vi "AM Modulation Demo (music) - Square.vi"() -> ()   [LabVIEW 2013]
uses:
  <vilib>/sound2/lvsound2.llb/Sound File Info (path).vi
  <vilib>/sound2/lvsound2.llb/Sound File Read Open.vi
  <vilib>/sound2/lvsound2.llb/Sound File Read (DBL).vi
  <vilib>/Waveform/WDTOps.llb/WDT Get Waveform Subset DBL.vi
  <vilib>/express/express analysis/Spectral/Block/exnSpectralBlock spectral measurements RMS poly.vi
  <vilib>/express/express analysis/Spectral/Block/exnSpectralBlock spectral measurements RMS DDT.vi
  <vilib>/express/express analysis/Spectral/Block/exnSpectralBlock spectral measurements power poly.vi
  <vilib>/express/express analysis/Spectral/Block/exnSpectralBlock spectral measurements power DDT.vi
  <vilib>/express/express analysis/Spectral/XNode/ExpressSpectralMeasurementsBlockNode.xnode
panel:
  in  "Duration":dbl
  in  "Path":path
  in  "WAV Sample Rate":dbl=44100.0 caption="dt"
  in  "Resample Rate.":dbl=2000.0 caption="Frequency"
  in  "LPF Cut-Off":dbl=10000.0 caption="Lower Cut-Off"
  in  "SNR (dB)":dbl(slide)=0.6 caption="Standard deviation" scale=-20.0..30.0
  out "Comparision":dynamicdata(graph)
  out "Baseband":dynamicdata(graph)
  out "DSB FFT":dynamicdata(graph)
  out "DSB Signal":dynamicdata(graph)
  out "?":dbl=1.0
  in  "Carrier Amp.":dbl=1.0 caption="Amplitude"
  in  "stop":bool
  in  "Frequency Offset":dbl(slide)=1.0 scale=0.0..1000.0
  in  "Carrier Freq.":dbl=100000.0 caption="Frequency"
  out "DSB Squared":dynamicdata(graph)=[{"t0"=timestamp(0 s since 1904-01-01), "dt"=10.0, "Y"=array[50000 elements], "attributes"=variant("NI_ChannelName"=variant(string "Sine (Power Spectrum)"), "NI_ExpIsRelativeTime"=variant(bool TRUE), "NI_ExpStartTimeStamp"=variant(timestamp timestamp(3635665779.2842293 s since 1904-01-01)), "NI_ExpTimeStamp"=variant(timestamp timestamp(3635665779.2842293 s since 1904-01-01)), "NI_ExpXDimension"=variant(string "f"), "NI_OriginalChannelName"=variant(string "Sine"))}]
  # "Amplitude Modulation"
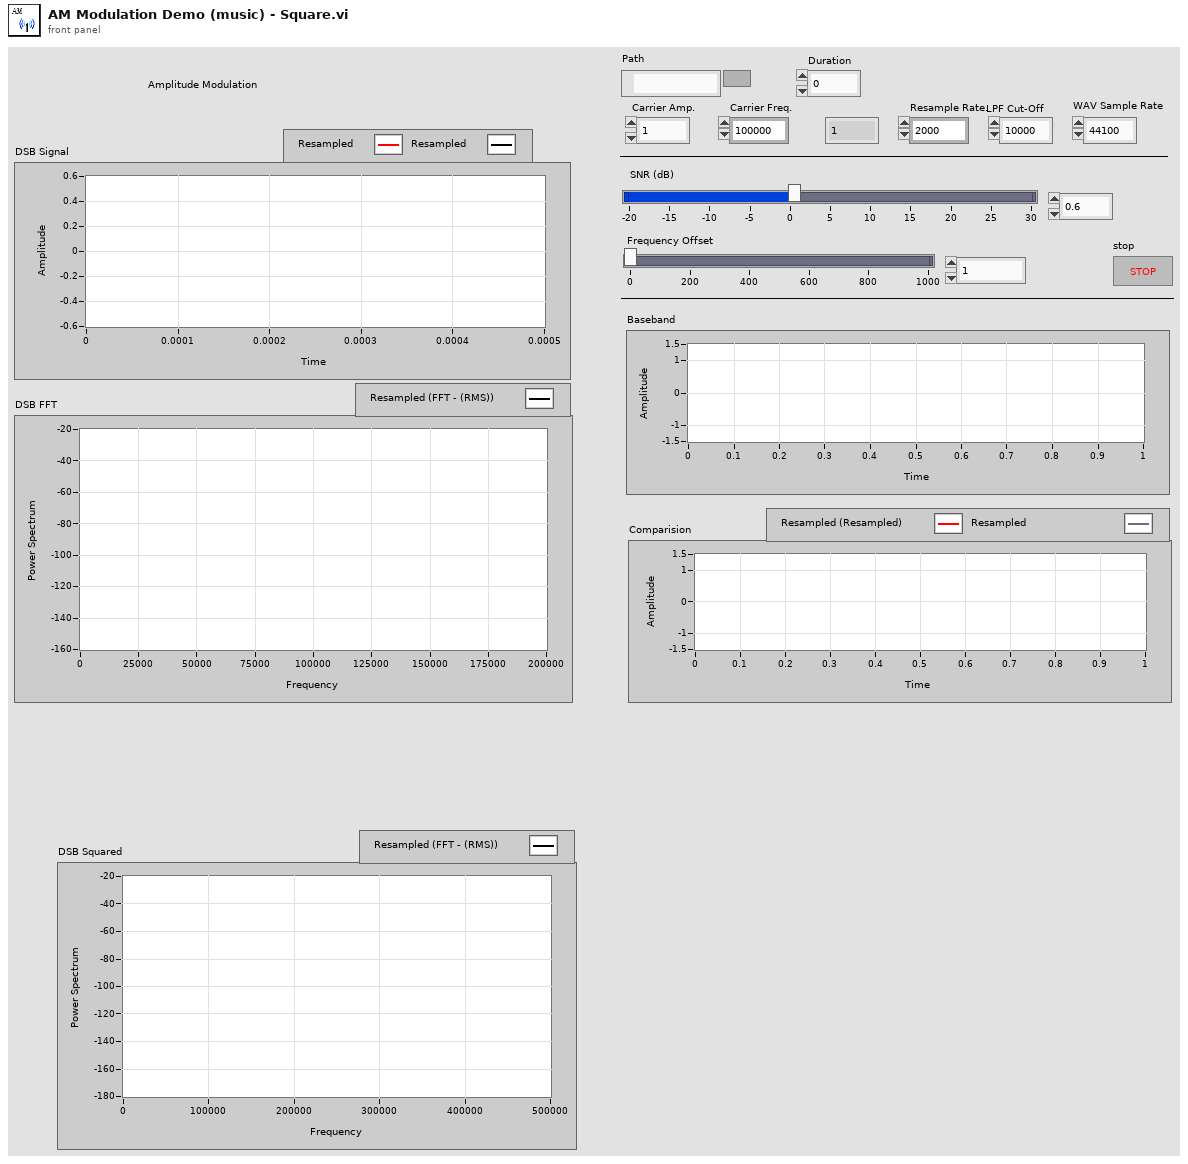
[diagram p1: front panel]
types:
  T1 = typedef "Sound File Refnum.ctl" = refnum<file>
  T2 = cluster{"averaging mode":u16, "weighting mode":u16, "number of averages":u32}
  T3 = cluster{"dB On (F)":bool, "unwrap phase (F)":bool, "convert to degree (F)":bool}
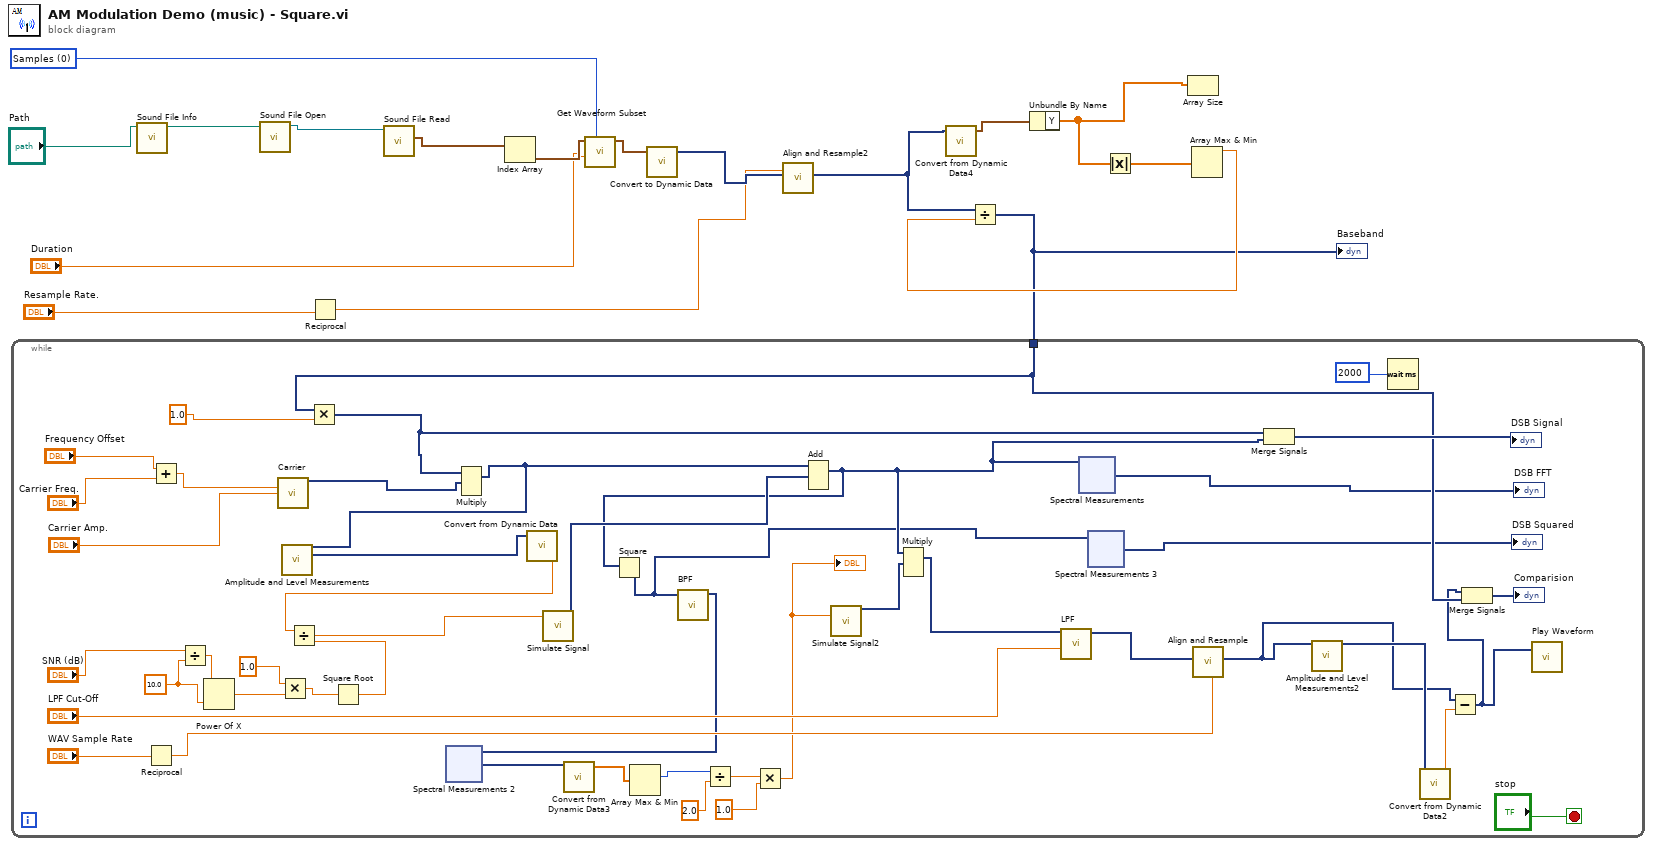
[diagram p0: block diagram]
diagram:
  w12 = u16 0 items=["Samples", "Relative Time"] ("start/duration format")
  n1 = call-poly <vilib>:"Sound File Info.vi"("path"="Path") -> ("path out"=w16:path)  [unwired: 7 in, 3 out]
  n2 = call-poly <vilib>:"Sound File Open.vi"("path"=w16) -> ("sound file refnum"=w15:T1)  [unwired: 9 in, 1 out]
  n3 = Reciprocal(x="Resample Rate.") -> (1/x=w7:dbl)
  n4 = call-poly <vilib>:"Sound File Read.vi"("sound file refnum"=w15) -> ("data"=w14:waveform(dbl)[])  [unwired: 6 in, 4 out]
  n5 = Index Array "Index Array"(array=w14) -> (element=w13:waveform(dbl))  [unwired: 1 in]
  n6 = call-poly <vilib>:"Get Waveform Subset.vi"("start/duration format"=w12, "duration"="Duration", "waveform in"=w13) -> ("waveform out"=w10:waveform(dbl))  [unwired: 3 in, 3 out]
  n7 = call "Convert to Dynamic Data"("Waveform"=w10) -> ("Dynamic Data Type"=w9:dynamicdata)  [unwired: 3 in]
  n8 = call "Align and Resample2"("dt"=w7, "Signals"=w9) -> ("Resampled Signals"=w3:dynamicdata)  [unwired: 7 in, 2 out]
  n9 = call "Convert from Dynamic Data4"("Dynamic Data Type"=w3) -> ("Waveform"=w6:waveform(dbl))  [unwired: 3 in]
  n10 = Unbundle By Name(w6) -> ("Y"=w5:dbl[])
  n11 = Absolute Value(x=w5) -> (abs(x)=w4:dbl[])
  n12 = Array Size(array=w5) -> ()  [unwired: 1 out]
  n13 = Array Max & Min(array=w4) -> (max value=w2:dbl)  [unwired: 3 out]
  n14 = Divide(x=w3, y=w2) -> (x/y=w1:dynamicdata)
  "Baseband" <- w1
  n15 = while {
    tunnel: w1 -> [w45]
    stop <- "stop" stop-if-true
    w41 = 10.0
    n16 = Reciprocal(x="WAV Sample Rate") -> (1/x=w49:dbl)
    n17 = Add(x="Frequency Offset", y="Carrier Freq.") -> (x+y=w34:dbl)
    n18 = Divide(x="SNR (dB)", y=w41) -> (x/y=w42:dbl)
    n19 = Power Of X(1:w41, 2:w42) -> (0:w40:dbl)
    n20 = call "Carrier"("Frequency"=w34, "Amplitude"="Carrier Amp.") -> ("Sine"=w61:dynamicdata)  [unwired: 12 in, 1 out]
    n21 = Multiply(x=1.0, y=w40) -> (x*y=w55:dbl)
    n22 = Multiply(x=w45, y=1.0) -> (x*y=w35:dynamicdata)
    n23 = Square Root(x=w55) -> (sqrt(x)=w53:dbl)
    n24 = Multiply(1:w61, 2:w35) -> (0:w52:dynamicdata)  [unwired: 1 in, 1 out]
    n25 = call "Amplitude and Level Measurements"("Signals"=w52) -> ("RMS"=w59:dynamicdata)  [unwired: 13 in, 1 out]
    n26 = call "Convert from Dynamic Data"("Dynamic Data Type"=w59) -> ("Scalar"=w54:dbl)  [unwired: 3 in]
    n27 = Divide(x=w54, y=w53) -> (x/y=w39:dbl)
    n28 = call "Simulate Signal"("Standard deviation"=w39) -> ("DC with Gaussian Noise"=w51:dynamicdata)  [unwired: 13 in, 1 out]
    n29 = Add(1:w51, 2:w52) -> (0:w28:dynamicdata)  [unwired: 1 in, 1 out]
    n30 = Square(x=w28) -> (x^2=w19:dynamicdata)
    n31 = call "BPF"("Signal"=w19) -> ("Filtered Signal"=w27:dynamicdata)  [unwired: 9 in, 1 out]
    n32 = xnode "Spectral Measurements 2"("Signals"=w27) -> ("Power Spectrum"=w26:dynamicdata)  [unwired: 1 in, 1 out]
    n33 = call "Convert from Dynamic Data3"("Dynamic Data Type"=w26) -> ("Array"=w25:dbl[])  [unwired: 3 in]
    n34 = Array Max & Min(array=w25) -> (max index (indices)=w24:i32)  [unwired: 3 out]
    n35 = Divide(x=w24, y=2.0) -> (x/y=w22:dbl)
    n36 = Multiply(x=w22, y=1.0) -> (x*y=w20:dbl)
    "?" <- w20
    n37 = call "Simulate Signal2"("Frequency"=w20) -> ("Sine"=w33:dynamicdata)  [unwired: 13 in, 1 out]
    n38 = Multiply(1:w33, 2:w28) -> (0:w32:dynamicdata)  [unwired: 1 in, 1 out]
    n39 = call "LPF"("Lower Cut-Off"="LPF Cut-Off", "Signal"=w32) -> ("Filtered Signal"=w48:dynamicdata)  [unwired: 8 in, 1 out]
    n40 = xnode "Spectral Measurements"("Signals"=w28) -> ("FFT - (RMS)"=→"DSB FFT":dynamicdata)  [unwired: 1 in, 2 out]
    n41 = xnode "Spectral Measurements 3"("Signals"=w19) -> ("FFT - (RMS)"=→"DSB Squared":dynamicdata)  [unwired: 1 in, 2 out]
    n42 = call "Align and Resample"("dt"=w49, "Signals"=w48) -> ("Resampled Signals"=w36:dynamicdata)  [unwired: 7 in, 2 out]
    n43 = Merge Signals(w35, w28) -> (→"DSB Signal":dynamicdata)
    n44 = call "Amplitude and Level Measurements2"("Signals"=w36) -> ("Mean (DC)"=w37:dynamicdata)  [unwired: 13 in, 1 out]
    n45 = Wait (ms)(milliseconds to wait=2000) -> ()  [unwired: 1 out]
    n46 = call "Convert from Dynamic Data2"("Dynamic Data Type"=w37) -> ("Scalar"=w44:dbl)  [unwired: 3 in]
    n47 = Subtract(x=w36, y=w44) -> (x-y=w38:dynamicdata)
    n48 = Merge Signals(w38, w45) -> (→"Comparision":dynamicdata)
    n49 = call "Play Waveform"("Data"=w38) -> ()  [unwired: 18 in, 1 out]
  }
